vi "step_read_hipot_V.vi"(8 "error in":errorcluster, 10 "step":T1 {"data num" format="%.3f"}) -> (0 "error out":errorcluster, 2 "Status":string)   [LabVIEW 2020]
uses:
  controls/step.ctl
  controls/step_type.ctl
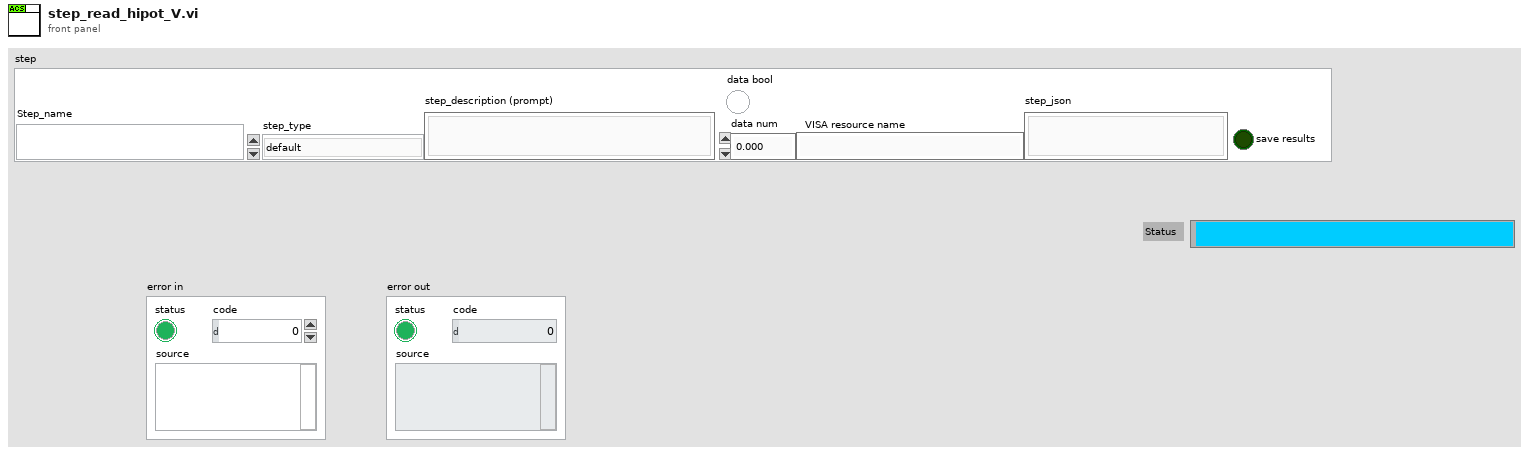
[diagram p1: front panel]
types:
  T1 = typedef "step.ctl" = cluster{"VISA resource name":string, "data num":dbl, "step_description (prompt)":string, "step_json":string, "save results":bool, "step_type":T2, "Step_name":string, "data bool":bool}
  T2 = typedef "step_type.ctl" = enum16{"default", "prompt", "sequence#", "12V power supply on_off", "set_hipot_V", "set_hipot_I_limit", "set_hipot_ramping (sec)", "set hipot_hold_time", "read_hipot_V", "read_hipot_I", "set_daq", "read_daq", "flash uds", "wait (sec)", "record_pass_fail", "stop_test", "error_exit"}
  T3 = cluster{"error":bool, "code":i8, "source":string}
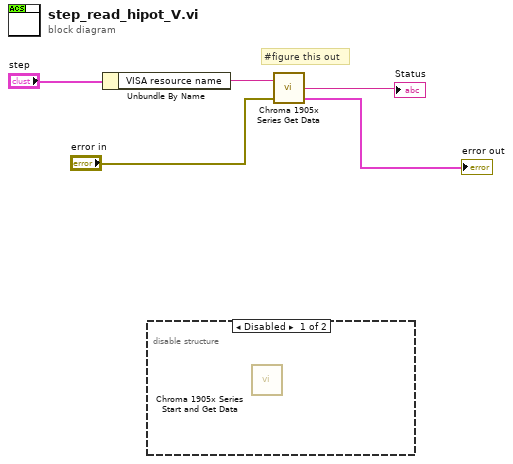
[diagram p0: block diagram]
diagram:
  # "#figure this out"
  n1 = Unbundle By Name("step") -> ("VISA resource name"=w5:string)
  n2 = disable-structure shown="Disabled" {
    frame Disabled {
      n3 = call <instrlib>:"Chroma 1905x Series Start and Get Data.vi"() -> ()  [unwired: 4 in, 6 out]
    }
    frame Enabled {
    }
  }
  n4 = call <instrlib>:"Chroma 1905x Series Get Data.vi"("inst handle in"=w5, "error in"="error in") -> ("Status"=→"Status":string, "error out"=→"error out":T3)  [unwired: 5 in, 1 out]
